vi "IpDFT.vi"(6 "IpDFT?":bool, 7 "FFT{X}":cxt[](array[numeric]), 9 "k0":i64, 10 "Nw":i32, 11 "Tw":dbl) -> (2 "X_stimata[f0]":cxt, 3 "f0 stimato":dbl)   [LabVIEW 2019]
panel:
  out "delta_stimato >=soglia?":bool
  in  "Soglia_delta_stimato":ext=1e-15
  out "alfa":ext
  out "x > y?":bool
  out "|Xw(k0-1)":ext
  out "|Xw(k0+1)|":ext
  out "delta_stimato":dbl
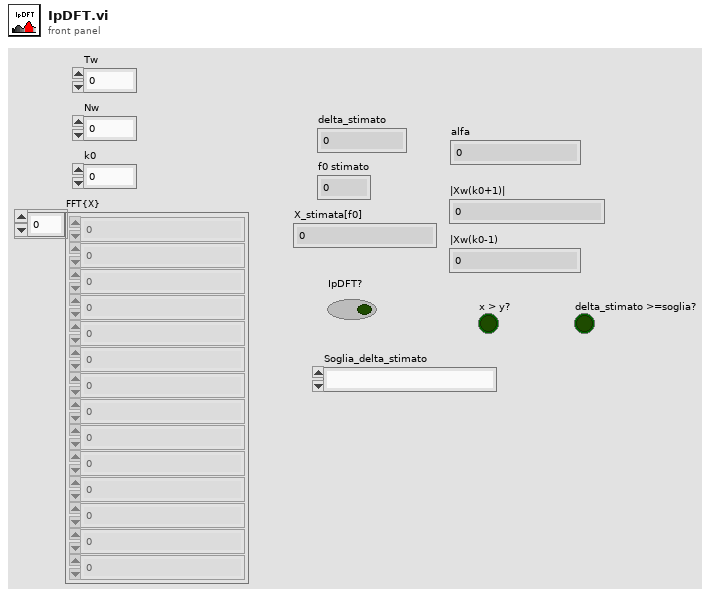
[diagram p1: front panel]
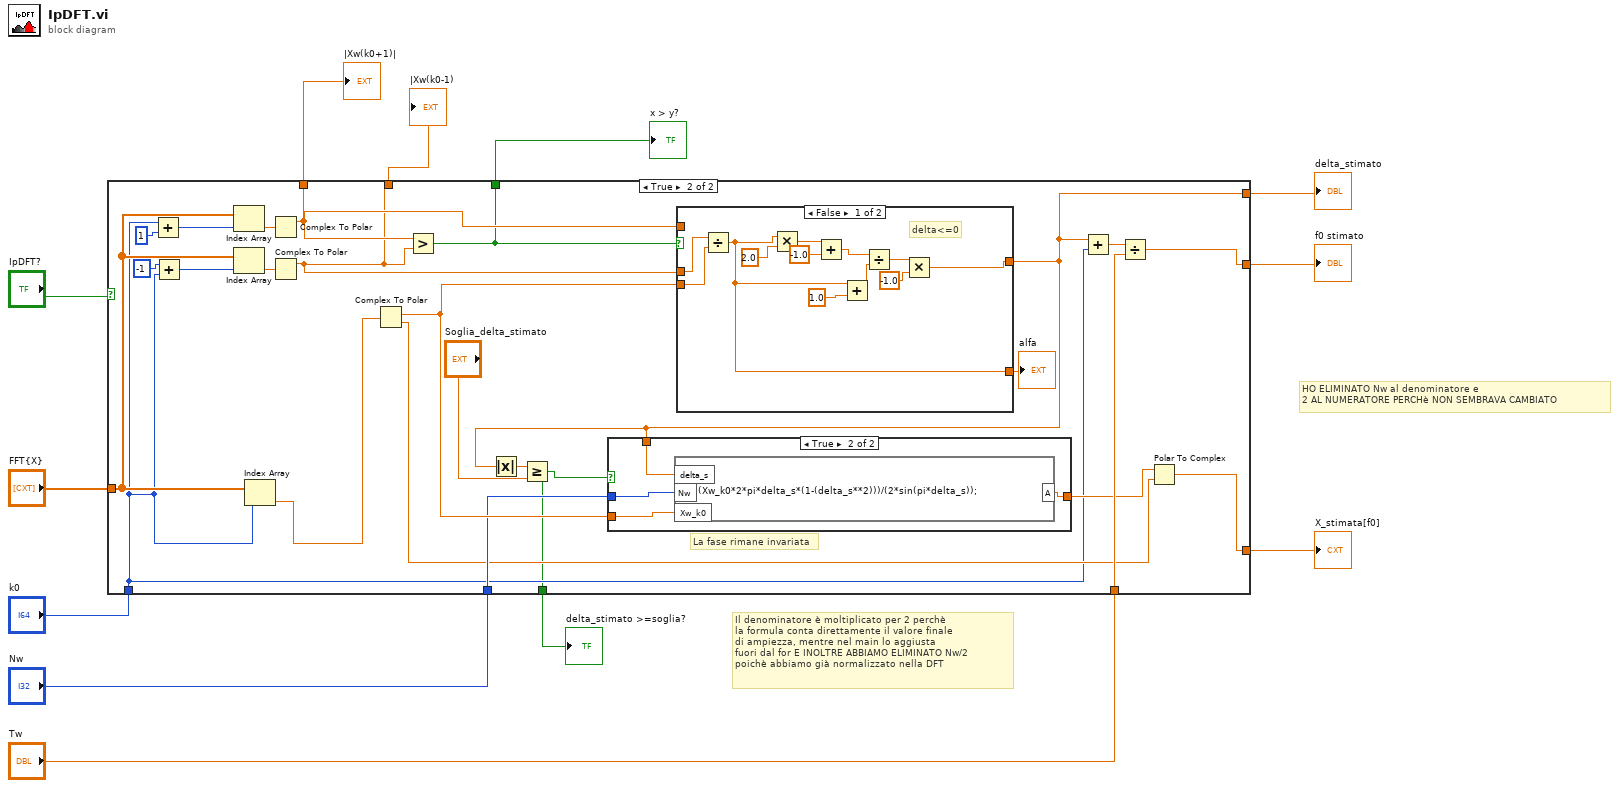
[diagram p0: block diagram]
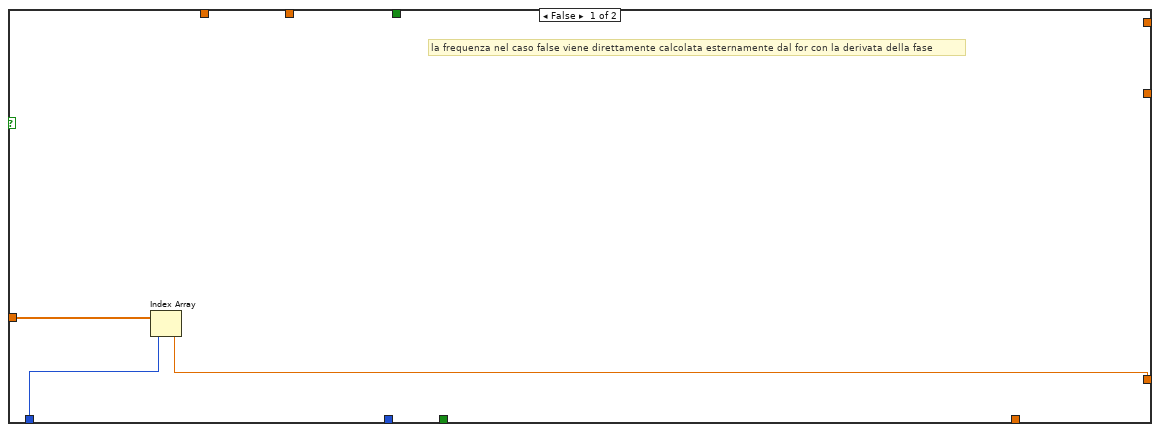
[diagram p2: hidden frame]
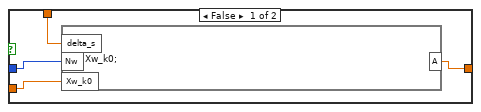
[diagram p3: hidden frame]
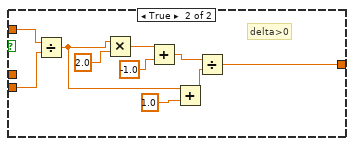
[diagram p4: hidden frame]
diagram:
  # "HO ELIMINATO Nw al denominatore e \n2 AL NUMERATORE PERCHè NON SEMBRAVA CAMBIATO"
  # "Il denominatore è moltiplicato per 2 perchè\nla formula conta direttamente il valore finale\ndi ampiezza, mentre nel main lo aggiusta\nfuori dal for E INOLTRE ABBIAMO ELIMINATO Nw/2 \npoichè abbiamo già normalizzato nella DFT"
  n1 = case shown="True" "IpDFT?" {
    tunnel: "FFT{X}" -> [w15 w37]
    tunnel: "k0" -> [w14 w24]
    tunnel: [w13 w26] -> w5
    tunnel: "Tw" -> [_ w33]
    tunnel: [_ w32] -> w6
    tunnel: "Nw" -> [_ w29]
    tunnel: [_ w17] -> w7
    tunnel: [_ w23] -> w4
    tunnel: [_ w22] -> w3
    tunnel: [_ w21] -> w2
    tunnel: [_ w16] -> w1
    frame False {
      # "la frequenza nel caso false viene direttamente calcolata esternamente dal for con la derivata della fase"
      n2 = Index Array(array=w15, index=w14) -> (element=w13:cxt)
    }
    frame True {
      # "La fase rimane invariata"
      n3 = Add(x=w24, y=i64 1) -> (x+y=w38:i64)
      n4 = Add(x=i64 -1 ("y"), y=w24) -> (x+y=w39:i64)
      n5 = Index Array(array=w37, index=w38) -> (element=w36:cxt)
      n6 = Index Array(array=w37, index=w39) -> (element=w35:cxt)
      n7 = Index Array(array=w37, index=w24) -> (element=w31:cxt)
      n8 = Complex To Polar(r * e^(i*theta)=w36) -> (r=w23:ext)  [unwired: 1 out]
      n9 = Complex To Polar(r * e^(i*theta)=w35) -> (r=w22:ext)  [unwired: 1 out]
      n10 = Complex To Polar(r * e^(i*theta)=w31) -> (r=w30:ext, theta=w28:ext)
      n11 = Greater?(x=w23, y=w22) -> (0:w21:bool)
      n12 = case shown="False" w21 {
        tunnel: w30 -> [w53 w69]
        tunnel: w22 -> [w54 _]
        tunnel: w23 -> [_ w70]
        tunnel: [w50 w61] -> w17
        tunnel: [w49 _] -> w20
        frame False {
          # "delta<=0"
          n13 = Divide(x=w54, y=w53) -> (x/y=w49:ext)
          n14 = Multiply(x=w49, y=2.0) -> (x*y=w59:ext)
          n15 = Add(x=w59, y=-1.0) -> (x+y=w57:ext)
          n16 = Add(x=w49, y=1.0) -> (x+y=w55:ext)
          n17 = Divide(x=w57, y=w55) -> (x/y=w52:ext)
          n18 = Multiply(x=w52, y=-1.0) -> (x*y=w50:ext)
        }
        frame True {
          # "delta>0"
          n19 = Divide(x=w70, y=w69) -> (x/y=w63:ext)
          n20 = Multiply(x=w63, y=2.0) -> (x*y=w67:ext)
          n21 = Add(x=w67, y=-1.0) -> (x+y=w65:ext)
          n22 = Add(x=w63, y=1.0) -> (x+y=w62:ext)
          n23 = Divide(x=w65, y=w62) -> (x/y=w61:ext)
        }
      }
      "alfa" <- w20
      n24 = Absolute Value(x=w17) -> (abs(x)=w18:ext)
      n25 = Greater Or Equal?(x=w18, y="Soglia_delta_stimato") -> (x >= y?=w16:bool)
      n26 = case shown="True" w16 {
        tunnel: w30 -> [w42 w48]
        tunnel: w29 -> [w44 w47]
        tunnel: [w41 w46] -> w27
        tunnel: w17 -> [w43 w45]
        frame False {
          n27 = formula code="A=Xw_k0;"("Xw_k0"=w42, "delta_s"=w43, "Nw"=w44) -> ("A"=w41:dbl)
        }
        frame True {
          n28 = formula code="A=(Xw_k0*2*pi*delta_s*(1-(delta_s**2)))/(2*sin(pi*delta_s));"("Xw_k0"=w48, "delta_s"=w45, "Nw"=w47) -> ("A"=w46:dbl)
        }
      }
      n29 = Add(x=w17, y=w24) -> (x+y=w34:ext)
      n30 = Divide(x=w34, y=w33) -> (x/y=w32:ext)
      n31 = Polar To Complex(1:w28, 2:w27) -> (0:w26:cxt)
    }
  }
  "X_stimata[f0]" <- w5
  "f0 stimato" <- w6
  "delta_stimato" <- w7
  "|Xw(k0+1)|" <- w4
  "|Xw(k0-1)" <- w3
  "x > y?" <- w2
  "delta_stimato >=soglia?" <- w1
